vi "DriveToTarget.vi"(8 "error in":errorcluster) -> (0 "error out":errorcluster)   [LabVIEW 2016]
uses:
  Robot Global Data.vi
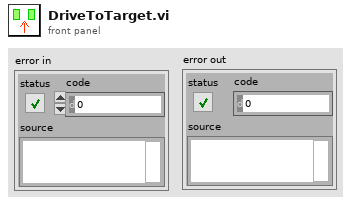
[diagram p1: front panel]
types:
  T1 = cluster{"Lower X":dbl, "Lower Y":dbl, "Upper X":dbl, "Upper Y":dbl}
  T2 = cluster{"Target?":bool, "Angle":dbl, "Distance":dbl}
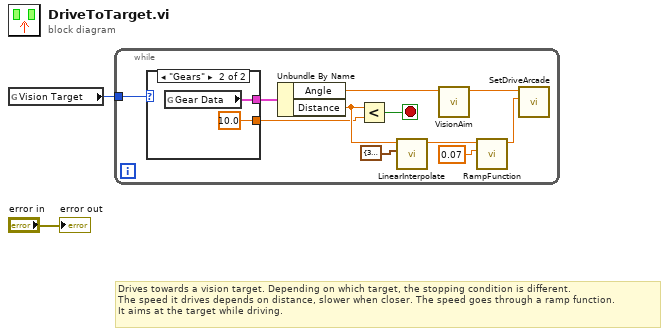
[diagram p0: block diagram]
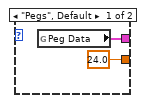
[diagram p2: hidden frame]
diagram:
  # "Drives towards a vision target. Depending on which target, the stopping condition is different.\nThe speed it drives depends on distance, slower when closer. The speed goes through a ramp function.\nIt aims at the target while driving."
  n1 = global read "Robot Global Data.vi" "Vision Target"() -> (w1:enum16{"Pegs", "Gears"})
  n2 = while {
    tunnel: w1 -> [w13]
    stop <- w7 stop-if-true
    n3 = case shown="\"Gears\"" w13 {
      tunnel: [w15 w17] -> w12
      tunnel: [24.0 ("y") 10.0 ("y")] -> w6
      frame "Pegs", Default {
        n4 = global read "Robot Global Data.vi" "Peg Data"() -> (w15:T2)
      }
      frame "Gears" {
        n5 = global read "Robot Global Data.vi" "Gear Data"() -> (w17:T2)
      }
    }
    n6 = Unbundle By Name(w12) -> ("Angle"=w11:dbl, "Distance"=w8:dbl)
    n7 = Less?(x=w8, y=w6) -> (x < y?=w7:bool)
    n8 = call "LinearInterpolate.vi"("Config"=T1 {"Lower X"=30.0, "Lower Y"=0.4, "Upper X"=60.0, "Upper Y"=0.75}, "Value"=w8) -> ("Output"=w4:dbl)  [unwired: 9 in]
    n9 = call "VisionAim.vi"("Angle"=w11) -> ("Turn"=w10:dbl)  [unwired: 9 in, 1 out]
    n10 = call "RampFunction.vi"("Max Rate"=0.07, "Input"=w4) -> ("Output"=w3:dbl)  [unwired: 9 in]
    n11 = call "SetDriveArcade.vi"("Forward"=w3, "Turn"=w10) -> ()  [unwired: 9 in, 1 out]
  }
  "error out" <- "error in"
